vi "StateMachine Example.vi"() -> ()   [LabVIEW 2012]
panel:
  out "Numeric":dbl
  in  "Array":dbl[](array[numeric])
  in  "Step":u32
  in  "Activate":bool
  in  "stop":bool
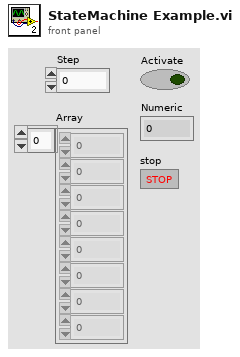
[diagram p1: front panel]
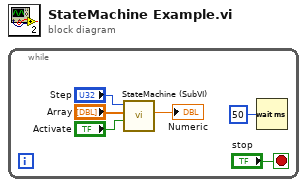
[diagram p0: block diagram]
diagram:
  n1 = while {
    stop <- "stop" stop-if-true
    n2 = call "StateMachine (SubVI).vi"("Activate"="Activate", "Array"="Array", "Step"="Step") -> ("Numeric"=→"Numeric":dbl)  [unwired: 8 in]
    n3 = Wait (ms)(milliseconds to wait=u32 50) -> ()  [unwired: 1 out]
  }
